vi "g_HCCConstants.vi"() -> ()   [LabVIEW 2014]
panel:
  out "HCC_NIL_Vsens_Y":dbl
  out "HCC_NIL_Vsens_X":dbl
  in  "HCC_VsenseRight_Y":dbl=1872.05
  in  "HCC_VsenseRight_X":dbl=2148.27
  out "HCC_NIL_GPO0_Y":dbl
  out "HCC_NIL_GPO0_X":dbl
  in  "HCC_GPO0_Y":dbl=1752.05
  in  "HCC_GPO0_X":dbl=711.7
  in  "HCC_NIL_BL_Y":dbl=4486.16
  in  "HCC_NIL_BL_X":dbl=2695.09
  in  "HCC_Width":dbl=2860.0
  in  "HCC_Length":dbl=4700.0
  # "HCC Constants (in micrometers)"
  # "Pad Locations"
  # "NIL Top Right"
  # "GPO0"
  # "VsenseRight"
  # "Distances"
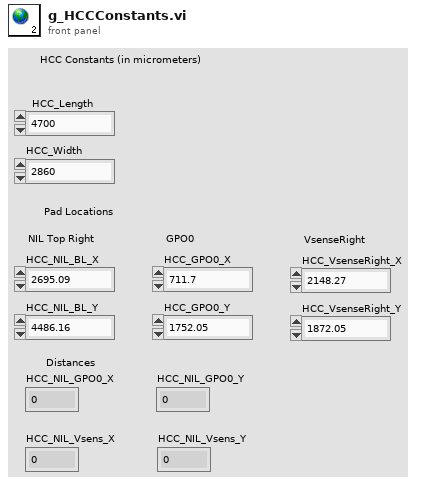
[diagram p1: front panel]
diagram:
